vi "CONTROLLO SOGLIE PRESSIONE.vi"(8 "Soglia minima\nassoluta":dbl=1.0, 9 "Soglia %":dbl, 10 "Set pressione":dbl, 11 "Pressione misurata":dbl) -> (1 "IN RANGE":bool, 2 "UP CONTROL":bool, 3 "DOWN CONTROL":bool)   [LabVIEW 2019]
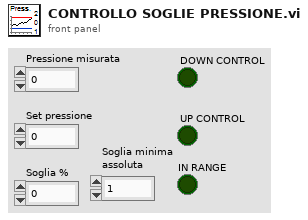
[diagram p1: front panel]
types:
  T1 = cluster{"DOWN CONTROL":bool, "UP CONTROL":bool}[]
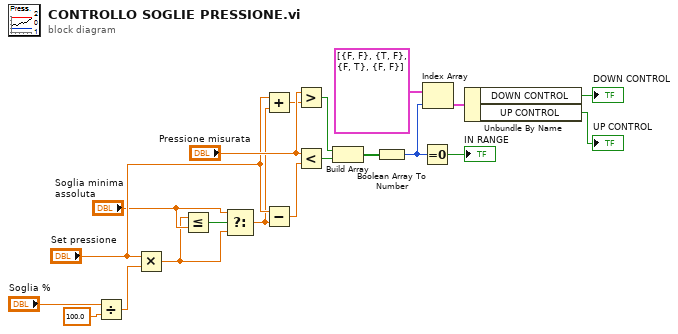
[diagram p0: block diagram]
diagram:
  n1 = Divide(x="Soglia %", y=100.0) -> (x/y=w9:dbl)
  n2 = Multiply(x="Set pressione", y=w9) -> (x*y=w2:dbl)
  n3 = Less Or Equal?(x=w2, y="Soglia minima\nassoluta") -> (x <= y?=w4:bool)
  n4 = Select(t="Soglia minima\nassoluta", s=w4, f=w2) -> (s? t:f=w1:dbl)
  n5 = Add(x="Set pressione", y=w1) -> (x+y=w11:dbl)
  n6 = Subtract(x="Set pressione", y=w1) -> (x-y=w13:dbl)
  n7 = Greater?(x="Pressione misurata", y=w11) -> (0:w14:bool)
  n8 = Less?(x="Pressione misurata", y=w13) -> (x < y?=w15:bool)
  n9 = Build Array(w14, w15) -> (w16:bool[])
  n10 = Boolean Array To Number(Boolean array=w16) -> (number=w6:u32)
  n11 = Equal To 0?(x=w6) -> (x = 0?=→"IN RANGE":bool)
  n12 = Index Array(array=T1 [{"DOWN CONTROL"=FALSE, "UP CONTROL"=FALSE}, {"DOWN CONTROL"=TRUE, "UP CONTROL"=FALSE}, {"DOWN CONTROL"=FALSE, "UP CONTROL"=TRUE}, {"DOWN CONTROL"=FALSE, "UP CONTROL"=FALSE}], index=w6) -> (element=w18:cluster{"DOWN CONTROL":bool, "UP CONTROL":bool})
  n13 = Unbundle By Name(w18) -> ("DOWN CONTROL"=→"DOWN CONTROL":bool, "UP CONTROL"=→"UP CONTROL":bool)
